vi "PIO Read Transfer Size Comparison.vi"() -> ()   [LabVIEW 2016]
uses:
  <vilib>/Platform/TimedLoop/XDataNode/timing_clust.ctl
  <vilib>/Platform/TimedLoop/XDataNode/nitl_modes.ctl
  <vilib>/Platform/TimedLoop/XDataNode/wakeup.ctl
  Source/GE 5565PIORC/GE 5565PIORC.lvclass/GE 5565PIORC.ctl
  <vilib>/Instr/_visa.llb/VISA Register Access Address Space.ctl
  Source/GE 5565PIORC/VIs/Registers/Local Configuration.LAS1RR.Address Range.Get.vi
  Source/GE 5565PIORC/VIs/Registers/Local Configuration.Get Register Offset.vi
  Source/GE 5565PIORC/GE 5565PIORC.lvclass
  <vilib>/platform/TimedLoop/XDataNode/XDataNode.xnode
  <vilib>/Platform/TimedLoop/XDataNode/XDNodeRunTimeDep.lvlib
panel:
  out "U64 Duration":dbl
  out "U32 Duration":dbl
  in  "Iterations":i32=1000
  out "U16 Duration":dbl
  in  "Bytes":i32=1024
  out "U8 Duration":dbl
  in  "VISA resource name":refnum<visa-resource-name>
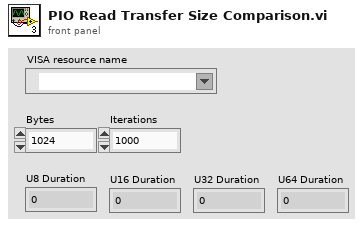
[diagram p1: front panel]
types:
  T1 = typedef "XDNodeRunTimeDep.lvlib/timing_clust.ctl" = cluster{"Expected End [f-1]":u64, "Actual End [f-1]":u64, "Finished Late? [f-1]":bool, "Expected End [i-1]":u64, "Actual End [i-1]":u64, "Finished Late? [i-1]":bool, "Expected Start [i]":u64, "Actual Start [i]":u64, "Expected Start [f]":u64, "Actual Start [f]":u64, "Source Name":string, "Structure Name":string, "Period":i64, "Deadline":i64, "Offset":i64, "Start":i64, "Priority":i32, "Timeout":i32, "Mode":T2, "Wakeup Reason":T3, "Error":errorcluster, "Source Type":string, "Secondary Source Type":string, "Global End Time":u64, "Global Start Time":u64, "Frame Duration":u64, "Iteration Duration":u64, "Assigned CPU":i32, "I/O Scan Engine Mode":u32}
  T2 = typedef "XDNodeRunTimeDep.lvlib/nitl_modes.ctl" = enum32{"No Change", "Process missed periods, maintain original phase", "Discard missed periods, maintain original phase", "Process missed periods, ignore original phase", "Discard missed periods, ignore original phase"}
  T3 = typedef "XDNodeRunTimeDep.lvlib/wakeup.ctl" = enum32{"Normal", "Aborted", "Asynchronous wakeup", "Timing source error", "Timed loop error", "Timeout"}
  T4 = typedef "VISA Register Access Address Space.ctl" = u16
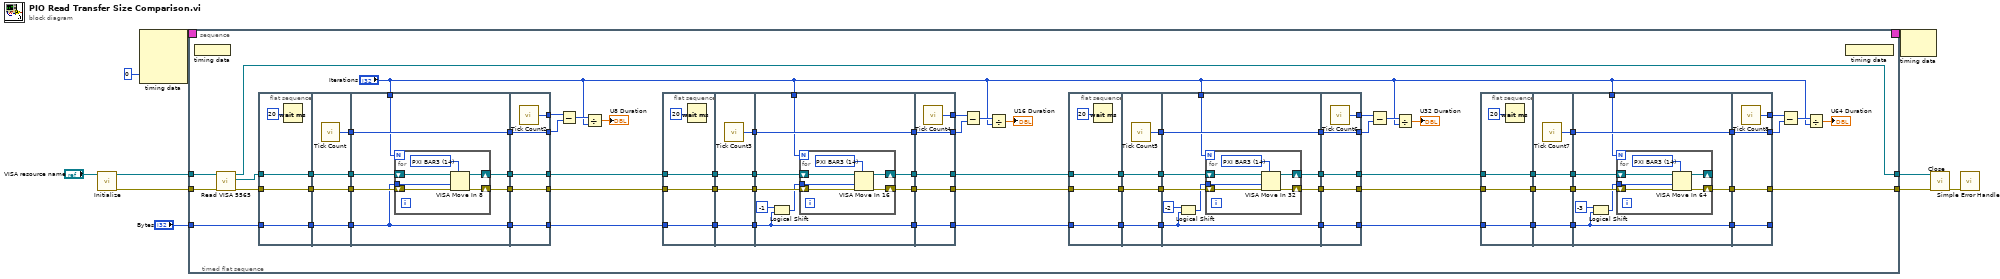
[diagram p0: block diagram]
diagram:
  n1 = call "Initialize.vi"("VISA resource name"="VISA resource name") -> ("error out"=w4:errorcluster, "GE 5565PIORC"=w5:refnum<class "GE 5565PIORC.lvclass">)  [unwired: 9 in]
  n2 = node-c288(0 ("Processor")) -> (w10:T1)  [unwired: 3 in]
  n3 = timed-sequence {
    timing: w10 -> [_]
    timing-out: [_] -> w9
    tunnel: w5 -> [w13]
    tunnel: w4 -> [w15]
    tunnel: "Bytes" -> [w14]
    tunnel: [w12] -> w2
    tunnel: [w11] -> w1
    n4 = timed-flat-sequence {
      tunnel: w15 -> [w77]
      tunnel: w14 -> [w82]
      tunnel: w13 -> [w78]
      tunnel: [w17] -> w12
      tunnel: [w16] -> w11
      n5 = node-c288() -> ()  [unwired: 1 in]
      n6 = call "Read VISA 5565.vi"("error in (no error)"=w77, "GE 5565PIORC in"=w78) -> ("error out"=w76:errorcluster, "VISA 5565"=w74:refnum<visa-resource-name>, "GE 5565PIORC out"=w16:refnum<class "GE 5565PIORC.lvclass">)  [unwired: 7 in]
      n7 = flat-sequence {
        tunnel: w76 -> [w176]
        tunnel: [w176] -> w86
        tunnel: w82 -> [w175]
        tunnel: [w175] -> w81
        tunnel: w74 -> [w174]
        tunnel: [w174] -> w73
        tunnel: [w181] -> w91
        tunnel: [w180] -> w87
        tunnel: w86 -> [w180]
        tunnel: w81 -> [w179]
        tunnel: [w179] -> w80
        tunnel: [w178] -> w75
        tunnel: w73 -> [w178]
        tunnel: w91 -> [w188]
        tunnel: [w188] -> w90
        tunnel: w87 -> [w186]
        tunnel: [w187] -> w85
        tunnel: w80 -> [w182]
        tunnel: [w182] -> w79
        tunnel: w75 -> [w185]
        tunnel: [w184] -> w72
        tunnel: "Iterations" -> [w183]
        tunnel: [w199] -> w89
        tunnel: [w198] -> w88
        tunnel: w90 -> [w198]
        tunnel: w85 -> [w195]
        tunnel: [w195] -> w55
        tunnel: w79 -> [w197]
        tunnel: [w197] -> w54
        tunnel: w72 -> [w196]
        tunnel: [w196] -> w56
        frame #0 {
          n8 = Wait (ms)(milliseconds to wait=u32 20) -> ()  [unwired: 1 out]
        }
        frame #1 {
          n9 = call "Tick Count"() -> ("Tick Count(uSec)"=w181:u32)
        }
        frame #2 {
          n10 = for {
            N: w183 -> [_]
            shift-right: [w191] -> w187
            shift-left: w186 -> [w192]
            shift-right: [w193] -> w184
            shift-left: w185 -> [w194]
            tunnel: w182 -> [w189]
            w190 = T4 14 items=["VXI/VME A16"=1, "VXI/VME A24"=2, "VXI/VME A32"=3, "VXI/VME A64"=4, "PXI Memory Allocations"=9, "PXI Configuration"=10, "PXI BAR0"=11, "PXI BAR1"=12, "PXI BAR2"=13, "PXI BAR3"=14, "PXI BAR4"=15, "PXI BAR5"=16] ("Address Space")
            n11 = VISA Move In 8(7:w190, 8:w192, 9:w189, 11:w194) -> (0:w191:errorcluster, 3:w193:refnum<visa-resource-name>)  [unwired: 1 in, 1 out]
          }
        }
        frame #3 {
          n12 = call "Tick Count2"() -> ("Tick Count(uSec)"=w199:u32)
        }
      }
      n13 = Subtract(x=w89, y=w88) -> (x-y=w84:u32)
      n14 = Divide(x=w84, y="Iterations") -> (x/y=→"U8 Duration":dbl)
      n15 = flat-sequence {
        tunnel: w55 -> [w148]
        tunnel: [w148] -> w71
        tunnel: w54 -> [w147]
        tunnel: [w147] -> w70
        tunnel: w56 -> [w146]
        tunnel: [w146] -> w69
        tunnel: [w153] -> w68
        tunnel: [w152] -> w67
        tunnel: w71 -> [w152]
        tunnel: w70 -> [w151]
        tunnel: [w151] -> w66
        tunnel: [w150] -> w65
        tunnel: w69 -> [w150]
        tunnel: w68 -> [w162]
        tunnel: [w162] -> w64
        tunnel: w67 -> [w160]
        tunnel: [w161] -> w63
        tunnel: w66 -> [w158]
        tunnel: [w158] -> w62
        tunnel: w65 -> [w159]
        tunnel: [w155] -> w61
        tunnel: "Iterations" -> [w154]
        tunnel: [w173] -> w60
        tunnel: [w172] -> w59
        tunnel: w64 -> [w172]
        tunnel: w63 -> [w171]
        tunnel: [w171] -> w37
        tunnel: w62 -> [w170]
        tunnel: [w170] -> w36
        tunnel: w61 -> [w169]
        tunnel: [w169] -> w38
        frame #0 {
          n16 = Wait (ms)(milliseconds to wait=u32 20) -> ()  [unwired: 1 out]
        }
        frame #1 {
          n17 = call "Tick Count3"() -> ("Tick Count(uSec)"=w153:u32)
        }
        frame #2 {
          n18 = Logical Shift(y=i16 -1, x=w158) -> (x << y=w156:i32)
          n19 = for {
            N: w154 -> [_]
            shift-right: [w165] -> w161
            shift-left: w160 -> [w166]
            shift-right: [w167] -> w155
            shift-left: w159 -> [w168]
            tunnel: w156 -> [w163]
            w164 = T4 14 items=["VXI/VME A16"=1, "VXI/VME A24"=2, "VXI/VME A32"=3, "VXI/VME A64"=4, "PXI Memory Allocations"=9, "PXI Configuration"=10, "PXI BAR0"=11, "PXI BAR1"=12, "PXI BAR2"=13, "PXI BAR3"=14, "PXI BAR4"=15, "PXI BAR5"=16] ("Address Space")
            n20 = VISA Move In 16(7:w164, 8:w166, 9:w163, 11:w168) -> (0:w165:errorcluster, 3:w167:refnum<visa-resource-name>)  [unwired: 1 in, 1 out]
          }
        }
        frame #3 {
          n21 = call "Tick Count4"() -> ("Tick Count(uSec)"=w173:u32)
        }
      }
      n22 = Subtract(x=w60, y=w59) -> (x-y=w58:u32)
      n23 = Divide(x=w58, y="Iterations") -> (x/y=→"U16 Duration":dbl)
      n24 = flat-sequence {
        tunnel: w37 -> [w120]
        tunnel: [w120] -> w53
        tunnel: w36 -> [w119]
        tunnel: [w119] -> w52
        tunnel: w38 -> [w118]
        tunnel: [w118] -> w51
        tunnel: [w125] -> w50
        tunnel: [w124] -> w49
        tunnel: w53 -> [w124]
        tunnel: w52 -> [w123]
        tunnel: [w123] -> w48
        tunnel: [w122] -> w47
        tunnel: w51 -> [w122]
        tunnel: w50 -> [w134]
        tunnel: [w134] -> w46
        tunnel: w49 -> [w132]
        tunnel: [w133] -> w45
        tunnel: w48 -> [w130]
        tunnel: [w130] -> w44
        tunnel: w47 -> [w131]
        tunnel: [w127] -> w43
        tunnel: "Iterations" -> [w126]
        tunnel: [w145] -> w42
        tunnel: [w144] -> w41
        tunnel: w46 -> [w144]
        tunnel: w45 -> [w143]
        tunnel: [w143] -> w20
        tunnel: w44 -> [w142]
        tunnel: [w142] -> w19
        tunnel: w43 -> [w141]
        tunnel: [w141] -> w21
        frame #0 {
          n25 = Wait (ms)(milliseconds to wait=u32 20) -> ()  [unwired: 1 out]
        }
        frame #1 {
          n26 = call "Tick Count5"() -> ("Tick Count(uSec)"=w125:u32)
        }
        frame #2 {
          n27 = Logical Shift(y=i16 -2, x=w130) -> (x << y=w128:i32)
          n28 = for {
            N: w126 -> [_]
            shift-right: [w137] -> w133
            shift-left: w132 -> [w138]
            shift-right: [w139] -> w127
            shift-left: w131 -> [w140]
            tunnel: w128 -> [w135]
            w136 = T4 14 items=["VXI/VME A16"=1, "VXI/VME A24"=2, "VXI/VME A32"=3, "VXI/VME A64"=4, "PXI Memory Allocations"=9, "PXI Configuration"=10, "PXI BAR0"=11, "PXI BAR1"=12, "PXI BAR2"=13, "PXI BAR3"=14, "PXI BAR4"=15, "PXI BAR5"=16] ("Address Space")
            n29 = VISA Move In 32(7:w136, 8:w138, 9:w135, 11:w140) -> (0:w137:errorcluster, 3:w139:refnum<visa-resource-name>)  [unwired: 1 in, 1 out]
          }
        }
        frame #3 {
          n30 = call "Tick Count6"() -> ("Tick Count(uSec)"=w145:u32)
        }
      }
      n31 = Subtract(x=w42, y=w41) -> (x-y=w40:u32)
      n32 = Divide(x=w40, y="Iterations") -> (x/y=→"U32 Duration":dbl)
      n33 = flat-sequence {
        tunnel: w20 -> [w94]
        tunnel: [w94] -> w35
        tunnel: w19 -> [w93]
        tunnel: [w93] -> w34
        tunnel: w21 -> [w92]
        tunnel: [w92] -> w33
        tunnel: [w99] -> w32
        tunnel: [w98] -> w31
        tunnel: w35 -> [w98]
        tunnel: w34 -> [w97]
        tunnel: [w97] -> w30
        tunnel: [w96] -> w29
        tunnel: w33 -> [w96]
        tunnel: w32 -> [w107]
        tunnel: [w107] -> w28
        tunnel: w31 -> [w105]
        tunnel: [w106] -> w27
        tunnel: w30 -> [w101]
        tunnel: [w101] -> w26
        tunnel: w29 -> [w104]
        tunnel: "Iterations" -> [w103]
        tunnel: [w117] -> w25
        tunnel: [w116] -> w24
        tunnel: w28 -> [w116]
        tunnel: w27 -> [w115]
        tunnel: [w115] -> w17
        tunnel: w26 -> [w114]
        tunnel: [w114] -> _
        frame #0 {
          n34 = Wait (ms)(milliseconds to wait=u32 20) -> ()  [unwired: 1 out]
        }
        frame #1 {
          n35 = call "Tick Count7"() -> ("Tick Count(uSec)"=w99:u32)
        }
        frame #2 {
          n36 = Logical Shift(y=i16 -3, x=w101) -> (x << y=w100:i32)
          n37 = for {
            N: w103 -> [_]
            shift-right: [w110] -> w106
            shift-left: w105 -> [w111]
            shift-right: [w112] -> _
            shift-left: w104 -> [w113]
            tunnel: w100 -> [w108]
            w109 = T4 14 items=["VXI/VME A16"=1, "VXI/VME A24"=2, "VXI/VME A32"=3, "VXI/VME A64"=4, "PXI Memory Allocations"=9, "PXI Configuration"=10, "PXI BAR0"=11, "PXI BAR1"=12, "PXI BAR2"=13, "PXI BAR3"=14, "PXI BAR4"=15, "PXI BAR5"=16] ("Address Space")
            n38 = VISA Move In 64(7:w109, 8:w111, 9:w108, 11:w113) -> (0:w110:errorcluster, 3:w112:refnum<visa-resource-name>)  [unwired: 1 in, 1 out]
          }
        }
        frame #3 {
          n39 = call "Tick Count8"() -> ("Tick Count(uSec)"=w117:u32)
        }
      }
      n40 = Subtract(x=w25, y=w24) -> (x-y=w23:u32)
      n41 = Divide(x=w23, y="Iterations") -> (x/y=→"U64 Duration":dbl)
      n42 = node-c288() -> ()  [unwired: 1 out]
    }
  }
  n43 = node-c288(w9) -> ()  [unwired: 1 out]
  n44 = call "Close.vi"("error in (no error)"=w2, "GE 5565PIORC in"=w1) -> ("error out"=w7:errorcluster)  [unwired: 8 in, 1 out]
  n45 = call <vilib>:"Simple Error Handler.vi"("error in (no error)"=w7) -> ()  [unwired: 4 in, 5 out]
